vi "Write Show UI.vi"(8 "error in (no error)":errorcluster, 10 "Applied Settings":bool, 11 "Settings UI in":refnum<class "Settings UI.lvclass">) -> (0 "error out":errorcluster, 3 "Settings UI out":refnum<class "Settings UI.lvclass">)   [LabVIEW 2020, in "Output Sequencer.lvlib" / "Settings UI.lvclass"]
uses:
  Settings UI.lvclass
  Settings UI.lvclass/Settings UI.ctl
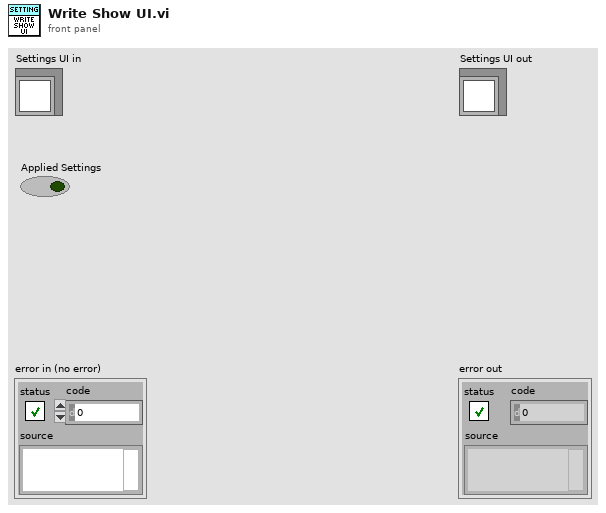
[diagram p1: front panel]
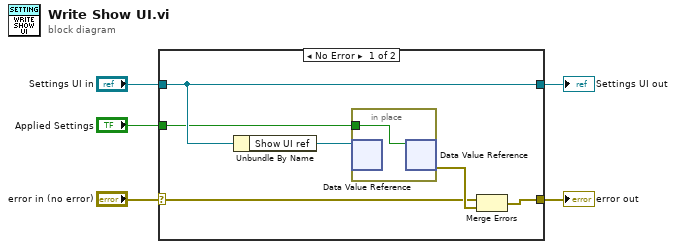
[diagram p0: block diagram]
diagram:
  n1 = case shown="No Error" "error in (no error)" {
    selector: "error in (no error)" -> [w7 w13]
    tunnel: [w6 w13] -> w4
    tunnel: [w9 w14] -> w2
    tunnel: "Settings UI in" -> [w9 w14]
    tunnel: "Applied Settings" -> [w8 _]
    frame No Error {
      n2 = Unbundle By Name(w9) -> ("Show UI ref"=w11:refnum<data-value>)
      n3 = in-place {
        in-place-border: w8 -> [w12]
        n4 = in-place-dvr #1(w11) -> ()  [unwired: 2 out]
        n5 = in-place-dvr #1(w12) -> (w10:errorcluster)  [unwired: 1 out]
      }
      n6 = Merge Errors(w7, w10) -> (w6:errorcluster)
    }
    frame Error {
    }
  }
  "error out" <- w4
  "Settings UI out" <- w2
